vi "AmpRamp.vi"(3 "Max step A":dbl, 4 "Desired current (A)":dbl, 5 "Actual Current":dbl[unit]) -> (0 "End Loop":bool, 2 "OutputCurrent":dbl[unit])   [LabVIEW 2017]
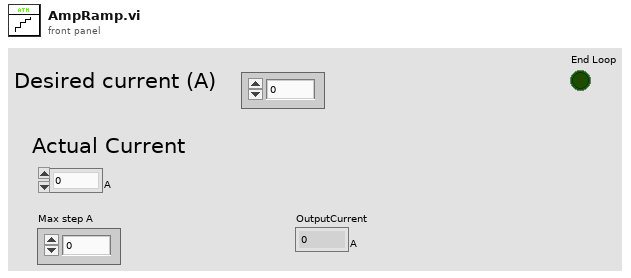
[diagram p1: front panel]
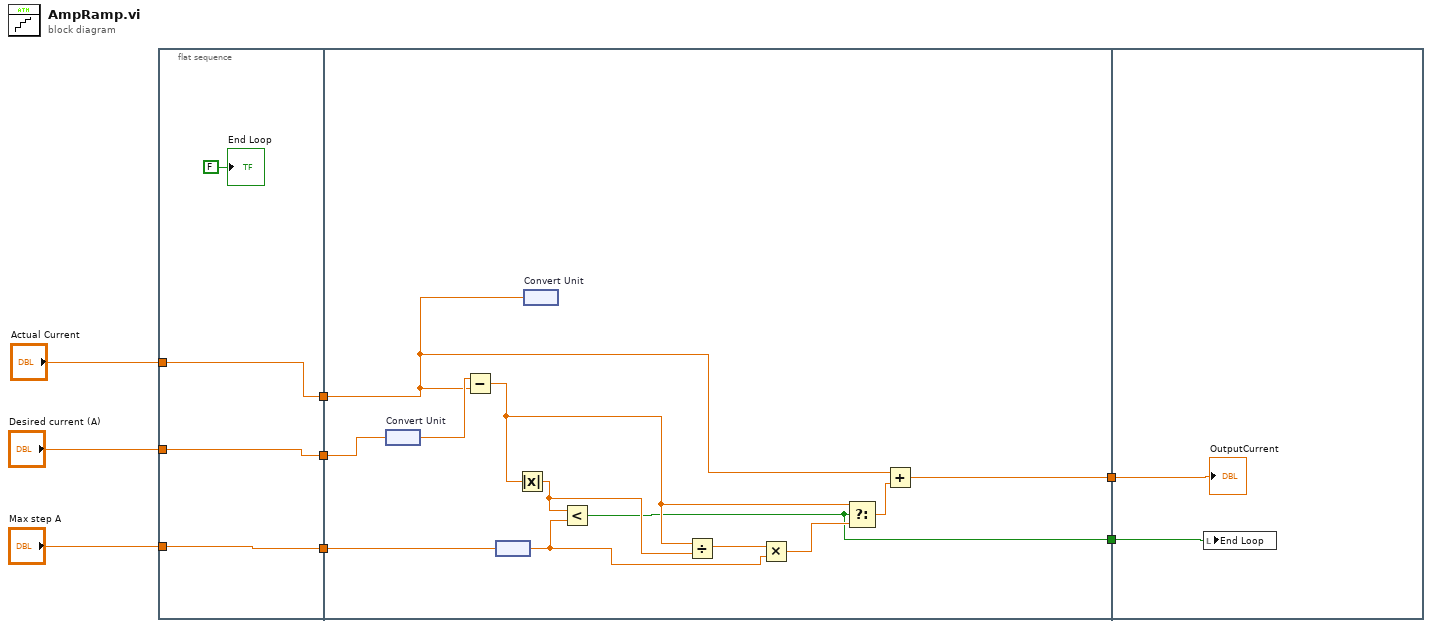
[diagram p0: block diagram]
diagram:
  n1 = flat-sequence {
    tunnel: [w11] -> w8
    tunnel: "Actual Current" -> [w11]
    tunnel: [w10] -> w6
    tunnel: "Desired current (A)" -> [w10]
    tunnel: "Max step A" -> [w9]
    tunnel: [w9] -> w1
    tunnel: w8 -> [w16]
    tunnel: w6 -> [w24]
    tunnel: [w15] -> w4
    tunnel: [w14] -> w3
    tunnel: w1 -> [w13]
    tunnel: w4 -> [w26]
    tunnel: w3 -> [w25]
    frame #0 {
      "End Loop" <- FALSE ("End Loop")
    }
    frame #1 {
      n2 = node "Convert Unit"(w24) -> (w17:dbl[unit])
      n3 = Subtract(x=w17, y=w16) -> (x-y=w19:dbl[unit])
      n4 = node(w13) -> (w21:dbl[unit])
      n5 = Absolute Value(x=w19) -> (abs(x)=w23:dbl[unit])
      n6 = node "Convert Unit"(w16) -> ()  [unwired: 1 out]
      n7 = Less?(x=w23, y=w21) -> (x < y?=w15:bool)
      n8 = Divide(x=w19, y=w23) -> (x/y=w22:dbl)
      n9 = Multiply(x=w22, y=w21) -> (x*y=w20:dbl[unit])
      n10 = Select(t=w19, s=w15, f=w20) -> (s? t:f=w18:dbl[unit])
      n11 = Add(x=w16, y=w18) -> (x+y=w14:dbl[unit])
    }
    frame #2 {
      n12 = local write "End Loop"(w26) -> ()
      "OutputCurrent" <- w25
    }
  }
